vi "Set Global Selector.vi"(8 "error in (no error)":errorcluster, 10 "Global Selector":bool, 11 "Item Ref in":T1 format="%.0x") -> (0 "error out":errorcluster)   [LabVIEW 2021, in "Software Multi-Plex System Explorer.lvlib"]
uses:
  Software Multi-Plex System Explorer.lvlib
  <vilib>/NI VeriStand/Custom Device API/Custom Device Item Ref.ctl
  Shared/Constants.vi
  <vilib>/NI VeriStand/Custom Device API/Set Item Property (Boolean).vi
  Shared/Software Multi-Plex Shared.lvlib
  <vilib>/NI VeriStand/Custom Device API/Custom Device API.lvlib
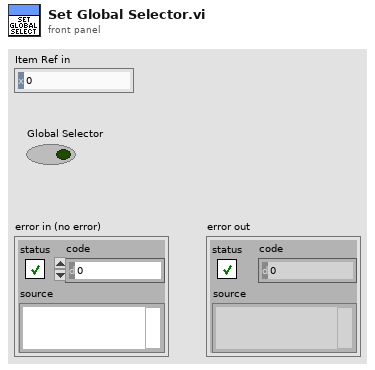
[diagram p1: front panel]
types:
  T1 = typedef "Custom Device API.lvlib/Custom Device Item Ref.ctl" = u64
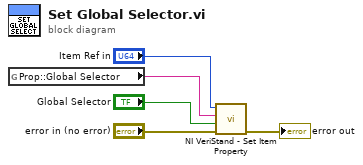
[diagram p0: block diagram]
diagram:
  n1 = global read "Constants.vi" "Prop::Global Selector"() -> (w3:string)
  n2 = call-poly <vilib>:"NI VeriStand - Set Item Property.vi"("error in (no error)"="error in (no error)", "Value"="Global Selector", "Property Name"=w3, "Item Ref in"="Item Ref in") -> ("error out"=→"error out":errorcluster)  [unwired: 5 in, 2 out]
